vi "FTW-Crypto-PublicKeySignature-Sign.vi"(0 "Data":string="Data to encrypt!", 5 "Private Key XML":string, 11 "error in":errorcluster) -> (4 "Hex Encoded Signature":string, 6 "Key Information":string, 15 "error out":errorcluster)   [LabVIEW 2015]
panel:
  # "Inputs"
  # "Outputs"
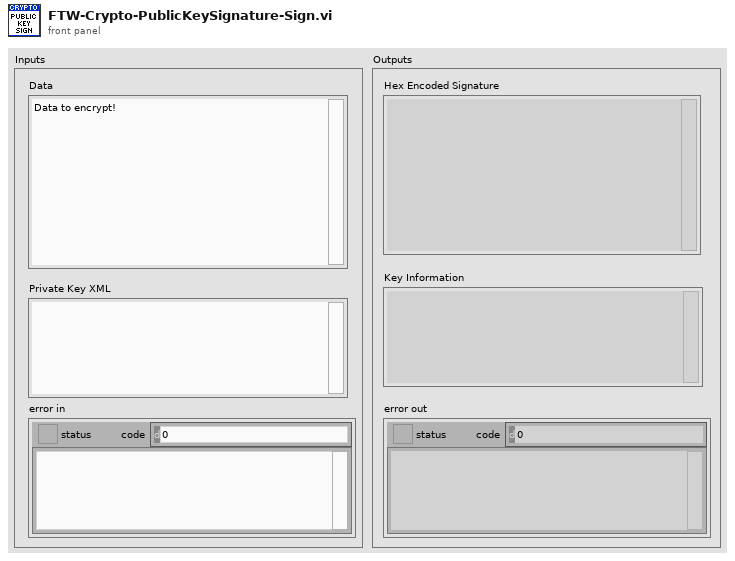
[diagram p1: front panel]
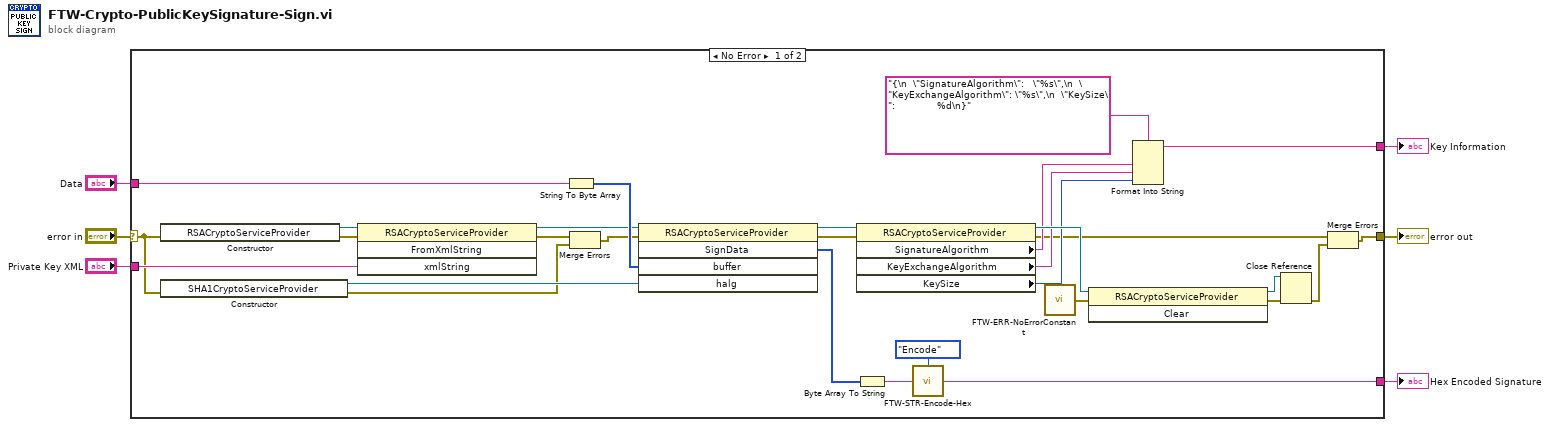
[diagram p0: block diagram]
diagram:
  n1 = case shown="No Error" "error in" {
    selector: "error in" -> [w19 w36]
    tunnel: "Data" -> [w34 _]
    tunnel: [w27 _] -> w5
    tunnel: "Private Key XML" -> [w30 _]
    tunnel: [w8 w36] -> w2
    tunnel: [w14 _] -> w1
    frame No Error {
      n2 = constructor class="RSACryptoServiceProvider"(error in=w19) -> (reference out=w31:refnum<k24>, error out=w32:errorcluster)  [unwired: 2 in, 1 out]
      n3 = constructor class="SHA1CryptoServiceProvider"(error in=w19) -> (reference out=w29:refnum<k24>, error out=w21:errorcluster)  [unwired: 2 in, 1 out]
      n4 = invoke class="RSACryptoServiceProvider" method="FromXmlString"(reference=w31, error in=w32, "xmlString"=w30) -> (reference out=w23:refnum<k24>, error out=w22:errorcluster)  [unwired: 1 in, 2 out]
      n5 = String To Byte Array(string=w34) -> (unsigned byte array=w33:u8[])
      n6 = Merge Errors(w22, w21) -> (w20:errorcluster)
      n7 = invoke class="RSACryptoServiceProvider" method="SignData"(reference=w23, error in=w20, "buffer"=w33, "halg"=w29) -> (reference out=w18:refnum<k24>, error out=w17:errorcluster, "SignData"=w35:u8[])  [unwired: 1 in, 2 out]
      n8 = property class="RSACryptoServiceProvider"(reference=w18, error in=w17) -> (reference out=w16:refnum<k24>, error out=w10:errorcluster, "SignatureAlgorithm"=w12:string, "KeyExchangeAlgorithm"=w11:string, "KeySize"=w13:i32)
      n9 = Byte Array To String(unsigned byte array=w35) -> (string=w28:string)
      n10 = call "FTW-STR-Encode-Hex.vi"("Input"=w28, "Direction"=enum16{"Encode", "Decode"}."Encode") -> ("Output"=w27:string)
      n11 = call "FTW-ERR-NoErrorConstant.vi"() -> ("no error"=w7:errorcluster)
      n12 = invoke class="RSACryptoServiceProvider" method="Clear"(reference=w16, error in=w7) -> (reference out=w24:refnum<k24>, error out=w25:errorcluster)  [unwired: 1 in, 1 out]
      n13 = Format Into String(format string="{\n  \"SignatureAlgorithm\":   \"%s\",\n  \"KeyExchangeAlgorithm\": \"%s\",\n  \"KeySize\":              %d\n}", w12, w11, w13) -> (resulting string=w14:string)  [unwired: 2 in, 1 out]
      n14 = Close Reference(reference=w24, error in (no error)=w25) -> (error out=w9:errorcluster)
      n15 = Merge Errors(w10, w9) -> (w8:errorcluster)
    }
    frame Error {
    }
  }
  "Hex Encoded Signature" <- w5
  "error out" <- w2
  "Key Information" <- w1
